vi "Bundle Script_Class Name to Clipboard.vi"(8 "error in":errorcluster, 11 "Affected Items":T1) -> (0 "error out":errorcluster)   [LabVIEW 2023]
doc: "Copy class name to clipboard."
uses:
  top/BundleMagic.ctl
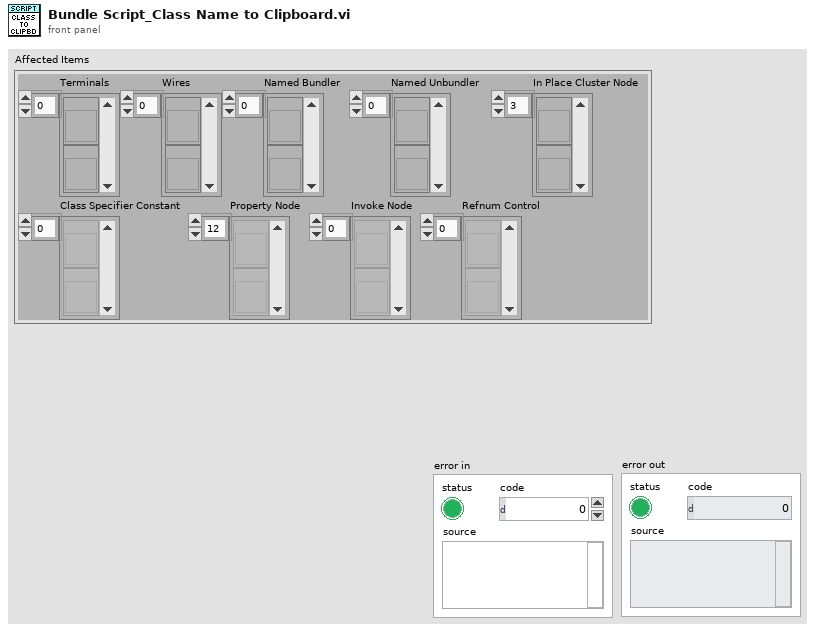
[diagram p1: front panel]
types:
  T1 = typedef "BundleMagic.ctl" = cluster{"Terminals":refnum<vi>[], "Wires":refnum<vi>[], "Named Bundler":refnum<vi>[], "Named Unbundler":refnum<vi>[], "In Place Cluster Node":refnum<vi>[], "Class Specifier Constant":refnum<vi>[], "Property Node":refnum<vi>[], "Invoke Node":refnum<vi>[], "Refnum Control":refnum<vi>[]}
  T2 = typedef "ASC_UniqueIDStringParentIDStringName.ctl" = cluster{"Unique ID string":string, "Parent ID string":string, "Class Name (unlocalized)":string, "Class Name (localized)":string}
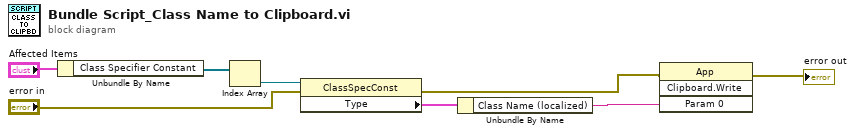
[diagram p0: block diagram]
diagram:
  n1 = Unbundle By Name("Affected Items") -> ("Class Specifier Constant"=w6:refnum<vi>[])
  n2 = Index Array(array=w6) -> (element=w7:refnum<vi>)  [unwired: 1 in]
  n3 = property class="ClassSpecConst"(reference=w7, error in="error in") -> (error out=w2:errorcluster, "Type"=w4:T2)  [unwired: 1 out]
  n4 = Unbundle By Name(w4) -> ("Class Name (localized)"=w3:string)
  n5 = invoke class="App" method="Clipboard.Write"(error in=w2, "Param 0"=w3) -> (error out=→"error out":errorcluster)  [unwired: 2 in, 3 out]
